vi "HW_GEN_Sync History Data FGV.vi"(10 "Data Blocks in":cluster{"Values":dbl[], "Timestamps":dbl[]}[](array[cluster]), 11 "Mode":enum16{"Get", "Set", "Init"}(ring)) -> (2 "Data Blocks out":cluster{"Values":dbl[], "Timestamps":dbl[]}[](array[cluster]))   [LabVIEW 2016]
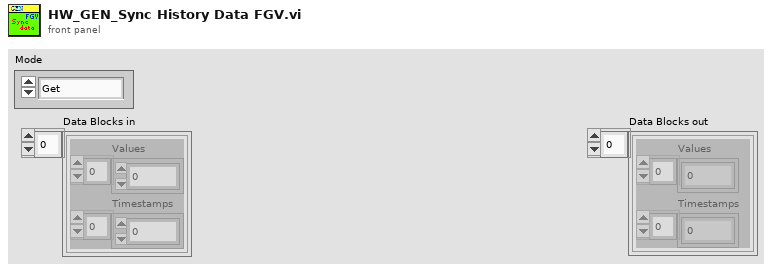
[diagram p1: front panel]
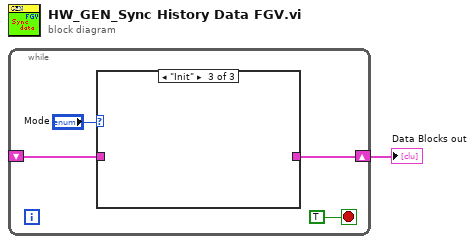
[diagram p0: block diagram]
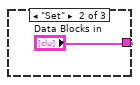
[diagram p3: hidden frame]
diagram:
  n1 = while {
    shift-right: [w3] -> w1
    shift-left: _ -> [w4]
    stop <- TRUE stop-if-true
    n2 = case shown="\"Init\"" "Mode" {
      tunnel: w4 -> [w6 _ _]
      tunnel: [w6 "Data Blocks in" _] -> w3
      frame "Get", Default {
      }
      frame "Set" {
      }
      frame "Init" {
      }
    }
  }
  "Data Blocks out" <- w1
